vi "Pos ctrl window-Mod state.vi"(3 "variant":variant, 4 "States":T2, 5 "Queue element in":T1) -> (2 "Modified queue element":T1)   [LabVIEW 2020]
uses:
  Typedefs/Pos Ctrl queue data cluster.ctl
  Typedefs/Pos Ctrl States.ctl
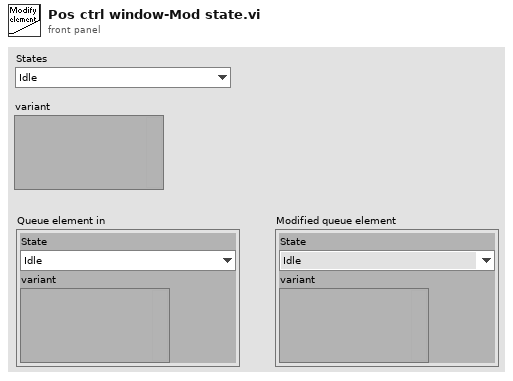
[diagram p1: front panel]
types:
  T1 = typedef "Pos Ctrl queue data cluster.ctl" = cluster{"State":T2, "variant":variant}
  T2 = typedef "Pos Ctrl States.ctl" = enum16{"Idle", "Count-down", "Request single step (ack.)", "Request single step (no ack.)", "Request continuous movement", "Request movement stop"}
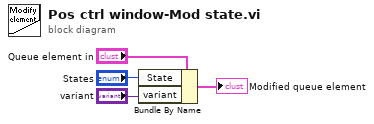
[diagram p0: block diagram]
diagram:
  n1 = Bundle By Name(cluster="Queue element in", "State"="States", "variant"="variant") -> (→"Modified queue element":T1)
